vi "Verify - Poly Fields Error.vi"(10 "Instance Info":T2={"VIPath"=path "C:/Projects/GitHub/data-record-ad-internal/Data Types/ADAS Generic/Read.vi", "Menu Name"="Generic", "Selector Name"="Generic"}, 11 "Poly Set":T1) -> (3 "Error":u32)   [LabVIEW 2020]
uses:
  _td_cluster_InstanceInfo.ctl
  _td_set_InstanceInfo.ctl
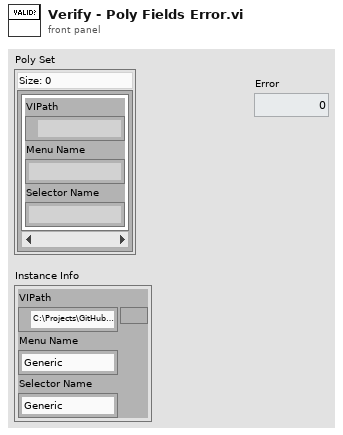
[diagram p1: front panel]
types:
  T1 = typedef "_td_set_InstanceInfo.ctl" = set{T2}
  T2 = typedef "_td_cluster_InstanceInfo.ctl" = cluster{"VIPath":path, "Menu Name":string, "Selector Name":string}
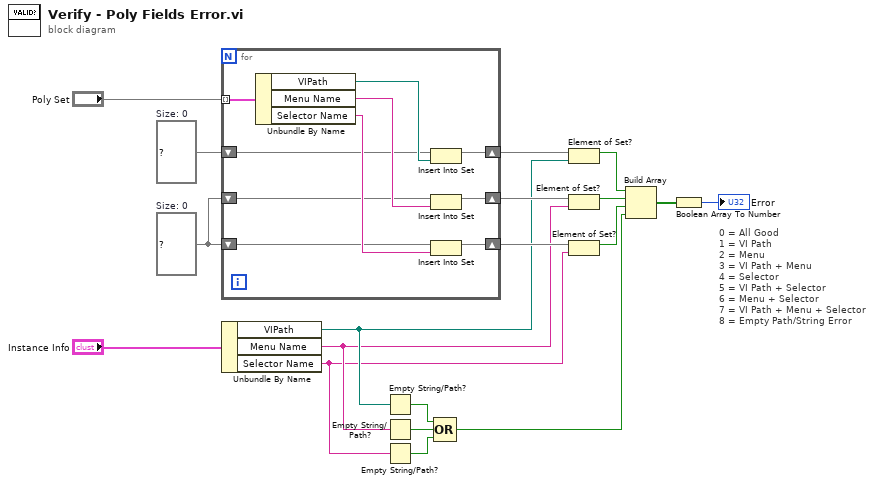
[diagram p0: block diagram]
diagram:
  w17 = set{string} {}  # Size: 0
  w18 = set{path} {}  # Size: 0
  # "0 = All Good\n1 = VI Path\n2 = Menu \n3 = VI Path + Menu \n4 = Selector \n5 = VI Path + Selector \n6 = Menu + Selector \n7 = VI Path + Menu + Selector\n8 = Empty Path/String Error"
  n1 = for {
    tunnel: "Poly Set" -> [w29] mode=indexing
    shift-right: [w25] -> w11
    shift-left: w18 -> [w24]
    shift-right: [w23] -> w9
    shift-left: w17 -> [w22]
    shift-right: [w21] -> w10
    shift-left: w17 -> [w20]
    n2 = Unbundle By Name(w29) -> ("VIPath"=w28:path, "Menu Name"=w27:string, "Selector Name"=w26:string)
    n3 = Insert Into Set(10:w28, 11:w24) -> (3:w25:set{path})  [unwired: 1 out]
    n4 = Insert Into Set(10:w27, 11:w22) -> (3:w23:set{string})  [unwired: 1 out]
    n5 = Insert Into Set(10:w26, 11:w20) -> (3:w21:set{string})  [unwired: 1 out]
  }
  n6 = Unbundle By Name("Instance Info") -> ("VIPath"=w7:path, "Menu Name"=w6:string, "Selector Name"=w5:string)
  n7 = Empty String/Path?(string/path=w7) -> (empty?=w4:bool)
  n8 = Empty String/Path?(string/path=w6) -> (empty?=w3:bool)
  n9 = Empty String/Path?(string/path=w5) -> (empty?=w2:bool)
  n10 = Compound Arithmetic op=OR(w4, w3, w2) -> (w1:bool)
  n11 = Element of Set?(10:w7, 11:w11) -> (3:w15:bool)
  n12 = Element of Set?(10:w6, 11:w9) -> (3:w14:bool)
  n13 = Element of Set?(10:w5, 11:w10) -> (3:w13:bool)
  n14 = Build Array(w15, w14, w13, w1) -> (w12:bool[])
  n15 = Boolean Array To Number(Boolean array=w12) -> (number=→"Error":u32)
